vi "Close.vi"(8 "error in (no error)":errorcluster, 11 "OPC UA in":refnum<class "OPC UA.lvclass">) -> (0 "error out":errorcluster, 3 "OPC UA out":refnum<class "OPC UA.lvclass">)   [LabVIEW 2021, in "OPC UA.lvclass"]
uses:
  OPC UA.lvclass
  OPC UA.lvclass/OPC UA.ctl
  <vilib>/OPCUA/NI OPC UA Client.lvlib
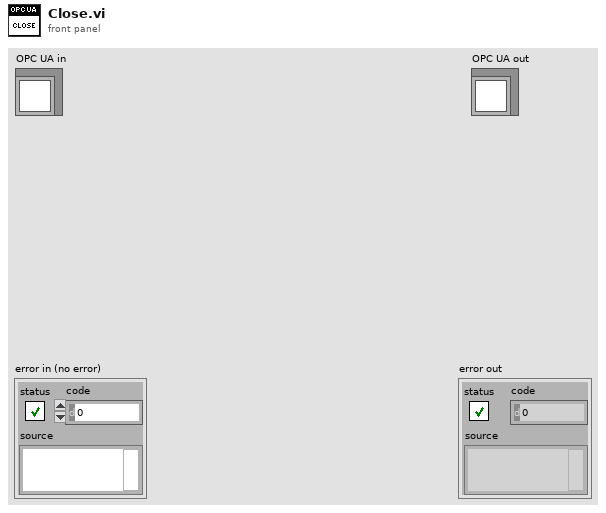
[diagram p1: front panel]
types:
  T1 = typedef "OPC UA Client Refnum.ctl" = refnum<k21>
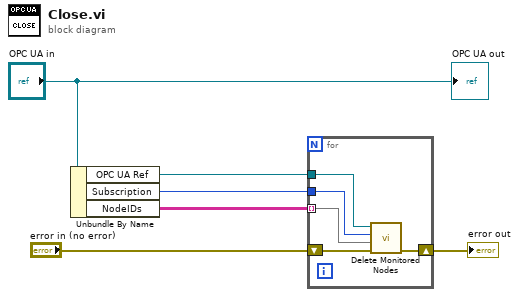
[diagram p0: block diagram]
diagram:
  n1 = Unbundle By Name("OPC UA in") -> ("OPC UA Ref"=w5:T1, "Subscription"=w4:u32, "NodeIDs"=w3:string[][])
  n2 = for {
    shift-right: [w11] -> w6
    shift-left: "error in (no error)" -> [w10]
    tunnel: w5 -> [w9]
    tunnel: w3 -> [w8] mode=indexing
    tunnel: w4 -> [w7]
    n3 = call <vilib>:"Delete Monitored Nodes.vi"("error in (no error)"=w10, "node IDs"=w8, "subscription ID in"=w7, "OPC UA client refnum in"=w9) -> ("error out"=w11:errorcluster)  [unwired: 3 in, 4 out]
  }
  "error out" <- w6
  "OPC UA out" <- "OPC UA in"
